vi "Write ScaledValue.vi"(8 "error in (no error)":errorcluster, 10 "ScaledValue":T1=1000000 items=["Bytes"=1, "KB"=1000, "MB"=1000000, "GB"=1000000000], 11 "HttpDownloadTask in":refnum<class "HttpDownloadTask.lvclass">) -> (0 "error out":errorcluster, 3 "HttpDownloadTask out":refnum<class "HttpDownloadTask.lvclass">)   [LabVIEW 2018, in "HttpClient_NET.lvlib" / "HttpDownloadTask.lvclass"]
uses:
  HttpDownloadTask.lvclass
  Types/ScaledValue_ring.ctl
  HttpDownloadTask.lvclass/HttpDownloadTask.ctl
  HttpClient_NET.lvlib
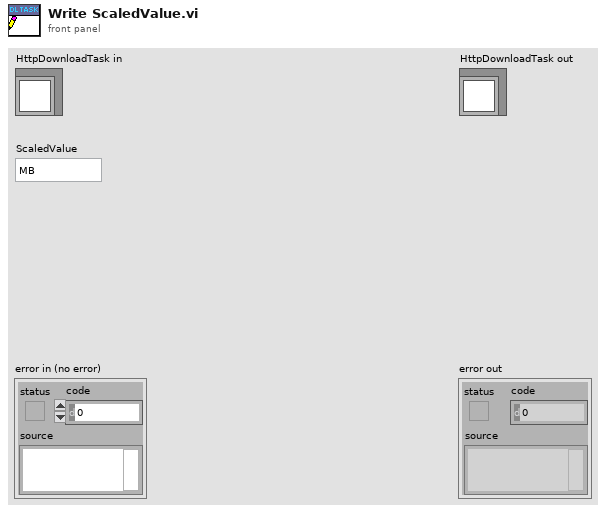
[diagram p1: front panel]
types:
  T1 = typedef "HttpClient_NET.lvlib/ScaledValue_ring.ctl" = u64
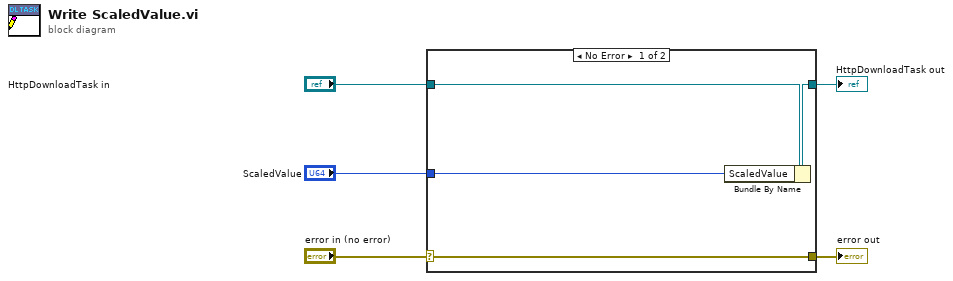
[diagram p0: block diagram]
diagram:
  n1 = case shown="No Error" "error in (no error)" {
    selector: "error in (no error)" -> [w9 w10]
    tunnel: [w9 w10] -> w4
    tunnel: [w7 w11] -> w2
    tunnel: "HttpDownloadTask in" -> [w8 w11]
    tunnel: "ScaledValue" -> [w6 _]
    frame No Error {
      n2 = Bundle By Name(cluster=w8, "ScaledValue"=w6) -> (w7:refnum<class "HttpDownloadTask.lvclass">)
    }
    frame Error {
    }
  }
  "error out" <- w4
  "HttpDownloadTask out" <- w2
